vi "KickForceIRL.vi"(0 "Game in":refnum<class "Game.lvclass">, 1 "KickValueTest":T1={"ForceValue"={"delta_kick"=0.0, "kick_min"=1.0, "kick_max"=0.0}, "BallValue"={"delta_ball"=0.0, "v_min_ball"=1.0, "v_max_ball"=0.0}, "Samples"=0.0, "Start"=FALSE, "id"=0, "RobotStopKick"=FALSE}, 3 "error in (no error)":errorcluster) -> (7 "Game out":refnum<class "Game.lvclass">, 8 "TestTeam":refnum<class "Ally.lvclass">, 10 "error out":errorcluster)   [LabVIEW 2021, in "Game.lvclass"]
uses:
  Game.lvclass
  Ally_class/Ally.lvclass
  KickValueTest/KickValuetest.ctl
  KickValueTest/KickValue.ctl
  KickValueTest/BallValue.ctl
  KickForceIRL/KickForceIRLstates.ctl
  Game.lvclass/Game.ctl
  Object_class/Object.lvclass/Object.ctl
  Ball_class/Ball.lvclass/Ball.ctl
  Team_class/Team.lvclass/Team.ctl
  RobotFeedback/RobotFeedback.lvclass/RobotFeedback.ctl
  Robot_class/Robot.lvclass/Robot.ctl
  RobotFeedback/Read id.vi
  RobotFeedback/Read dribblerContactToBall.vi
  <vilib>/Analysis/baseanly.llb/Unit Vector (DBL).vi
  Robot_class/Write kick_x.vi
  Robot_class/Write dest_x.vi
  Robot_class/Write dest_y.vi
  Read BallRef.vi
  Read FieldRef.vi
  Read AllyRef.vi
  Read Utilities.lvclass.vi
  Read TestTeam.vi
  Read RobotsFeedback.vi
  Team_class/Read RobotRef.vi
  Object_class/Read position(x,y).vi
  Ball_class/Read v_x.vi
  Ball_class/Read v_y.vi
  Object_class/Read x.vi
  Object_class/Read y.vi
  Team_class/Write RobotRef.vi
  Ball_class/Ball.lvclass
  Robot_class/Robot.lvclass
  <vilib>/Analysis/1siggen.llb/Ramp Pattern by Delta.vi
  Field_class/Field.lvclass
  Utilities_class/Utilities.lvclass
  RobotFeedback/RobotFeedback.lvclass
  <vilib>/Analysis/NI_AALBase.lvlib
panel:
  out "appended array":dbl[][](array[numeric])
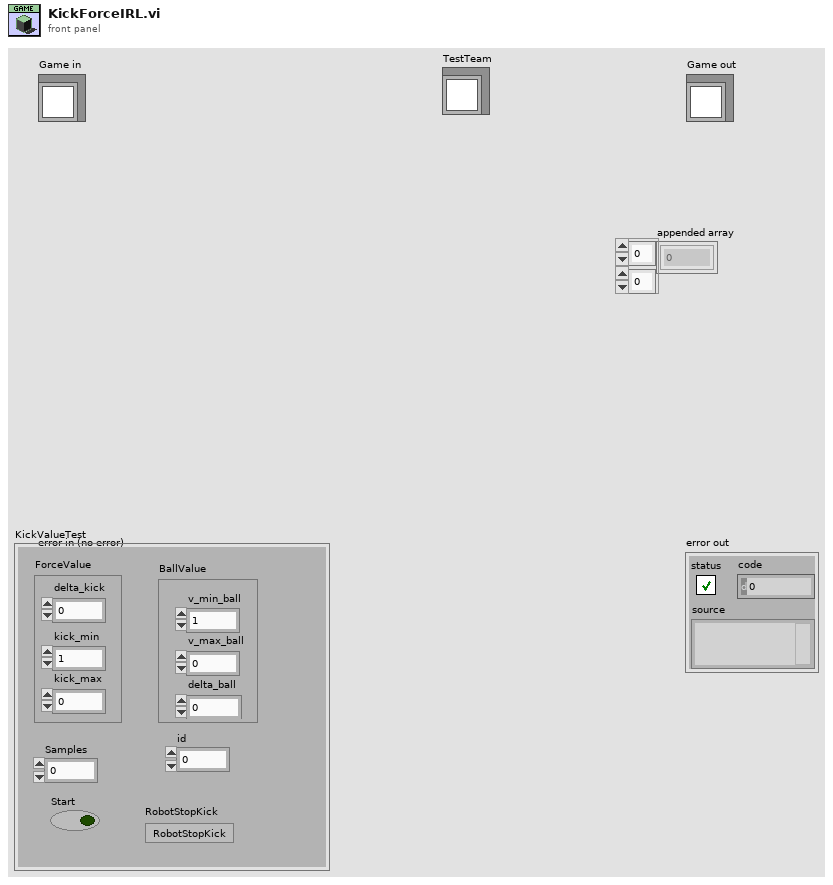
[diagram p1: front panel]
types:
  T1 = typedef "KickValuetest.ctl" = cluster{"ForceValue":T2, "BallValue":T3, "Samples":dbl, "Start":bool, "id":i32, "RobotStopKick":bool}
  T2 = typedef "Game.lvclass/KickValue.ctl" = cluster{"delta_kick":dbl, "kick_min":dbl, "kick_max":dbl}
  T3 = typedef "Game.lvclass/BallValue.ctl" = cluster{"delta_ball":dbl, "v_min_ball":dbl, "v_max_ball":dbl}
  T4 = typedef "Game.lvclass/KickForceIRLstates.ctl" = enum16{"Ball positioning", "Start count time", "Kicking ball", "Waiting ball v=0", "Saiving kick force, time and distance", "Finish"}
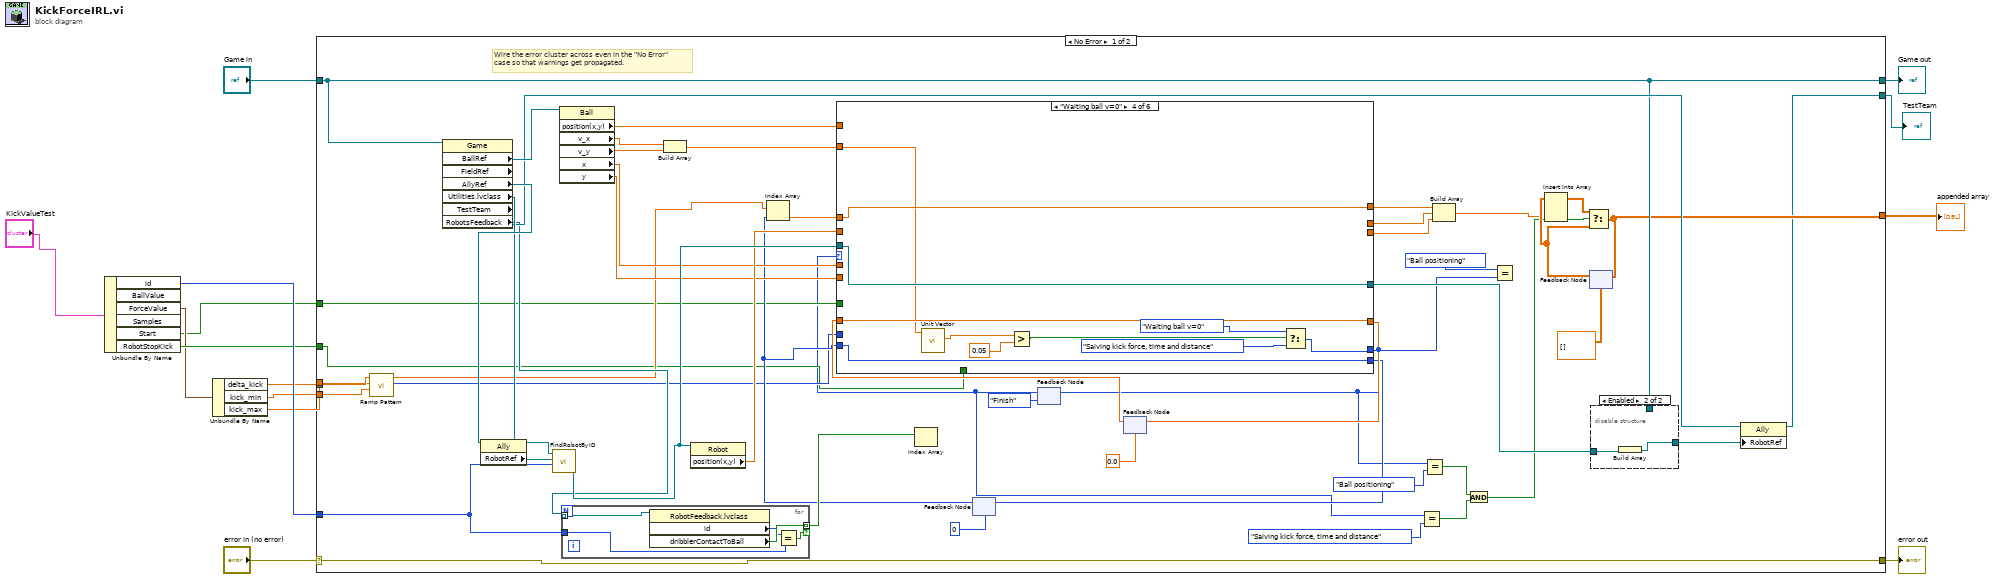
[diagram p0: block diagram]
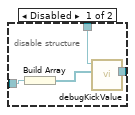
[diagram p2: hidden frame]
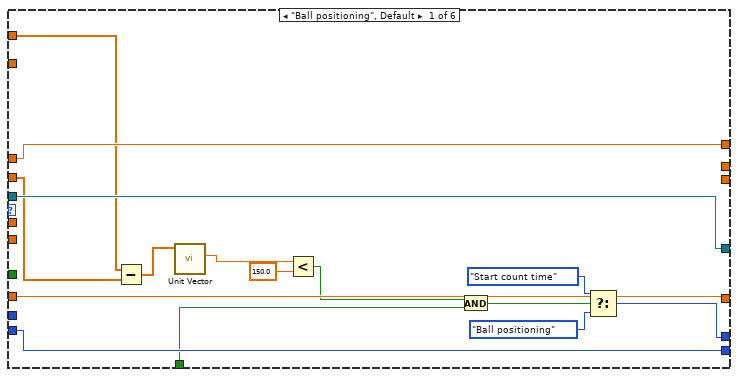
[diagram p3: hidden frame]
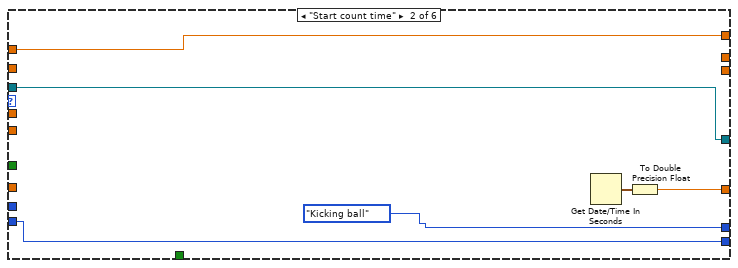
[diagram p4: hidden frame]
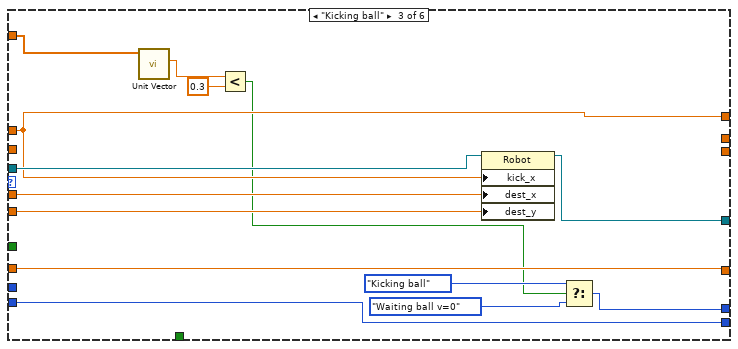
[diagram p5: hidden frame]
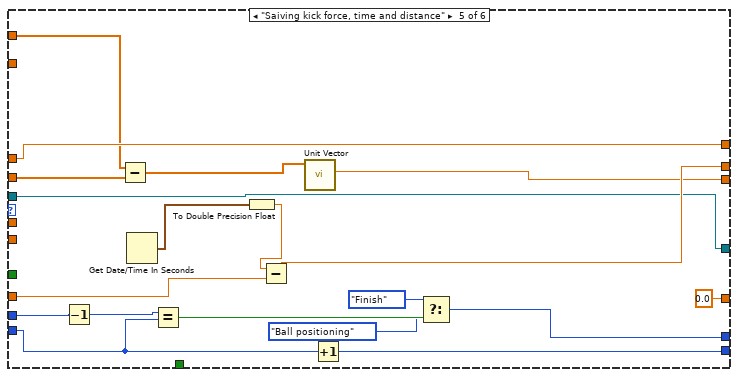
[diagram p6: hidden frame]
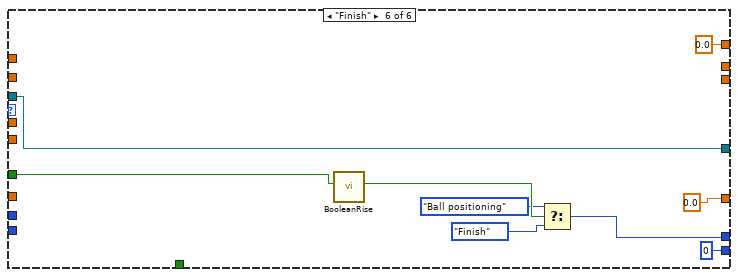
[diagram p7: hidden frame]
diagram:
  n1 = Unbundle By Name("KickValueTest") -> ("id"=w8:i32, "ForceValue"=w6:T2, "Start"=w2:bool, "RobotStopKick"=w7:bool)  [unwired: 2 out]
  n2 = Unbundle By Name(w6) -> ("delta_kick"=w5:dbl, "kick_min"=w4:dbl, "kick_max"=w3:dbl)
  n3 = case shown="No Error" "error in (no error)" {
    selector: "error in (no error)" -> [w66 w153]
    tunnel: [w66 w153] -> w13
    tunnel: [w59 w152] -> w11
    tunnel: "Game in" -> [w59 w152]
    tunnel: [w32 _] -> w10
    tunnel: w8 -> [w40 _]
    tunnel: w7 -> [w25 _]
    tunnel: [w42 _] -> w1
    tunnel: w5 -> [w36 _]
    tunnel: w4 -> [w35 _]
    tunnel: w3 -> [w34 _]
    tunnel: w2 -> [w28 _]
    frame No Error {
      # "Wire the error cluster across even in the \"No Error\"\ncase so that warnings get propagated."
      n4 = call-poly <vilib>:"Ramp Pattern.vi"("start"=w35, "end"=w34, "delta"=w36) -> ("samples"=w30:i32, "Ramp Pattern"=w29:dbl[])  [unwired: 6 in, 1 out]
      n5 = property class="Game" props=["BallRef", "FieldRef", "AllyRef", "Utilities.lvclass", "TestTeam", "RobotsFeedback"](reference=w59) -> ("BallRef"=w65:refnum<class "Ball.lvclass">, "AllyRef"=w64:refnum<class "Ally.lvclass">, "Utilities.lvclass"=w62:refnum<class "Utilities.lvclass">, "TestTeam"=w61:refnum<class "Ally.lvclass">, "RobotsFeedback"=w41:refnum<class "RobotFeedback.lvclass">[])  [unwired: 1 in, 3 out]
      n6 = property class="Ally"(reference=w64) -> ("RobotRef"=w63:refnum<class "Robot.lvclass">[])  [unwired: 1 in, 2 out]
      n7 = call "FindRobotByID.vi"("id"=w40, "RobotRef"=w63, "Utilities in"=w62) -> ("Robot"=w58:refnum<class "Robot.lvclass">)  [unwired: 5 in, 3 out]
      n8 = property class="Ball"(reference=w65) -> ("position(x,y)"=w45:dbl[], "v_x"=w51:dbl, "v_y"=w50:dbl, "x"=w38:dbl, "y"=w37:dbl)  [unwired: 1 in, 2 out]
      n9 = for {
        tunnel: w41 -> [w77] mode=indexing
        tunnel: w40 -> [w74]
        tunnel: [w76] -> w39 mode=indexing if=w73
        n10 = property class="RobotFeedback.lvclass"(reference=w77) -> ("id"=w75:i32, "dribblerContactToBall"=w76:bool)  [unwired: 1 in, 2 out]
        n11 = Equal?(x=w75, y=w74) -> (x = y?=w73:bool)
      }
      n12 = Build Array(w51, w50) -> (w49:dbl[])
      n13 = property class="Robot"(reference=w58) -> ("position(x,y)"=w46:dbl[])  [unwired: 1 in, 2 out]
      n14 = Index Array(array=w39) -> ()  [unwired: 1 in, 1 out]
      n15 = feedback #1(0) -> (w31:i32)
      n16 = Index Array(array=w29, index=w31) -> (element=w47:dbl)
      n17 = feedback #2(KickForceIRLstates."Finish" ("t")) -> (w21:T4)
      n18 = feedback #3(0.0) -> (w56:dbl)
      n19 = case shown="\"Waiting ball v=0\"" w21 {
        tunnel: [w78 KickForceIRLstates."Kicking ball" w103 w117 w129 w143] -> w24
        tunnel: [w92 w96 w112 w123 0.0 0.0] -> w57
        tunnel: w56 -> [w92 _ w112 w123 w142 _]
        tunnel: [_ _ _ _ w139 _] -> w55
        tunnel: w58 -> [w89 w93 w111 w115 w133 w150]
        tunnel: [w91 w95 w110 w122 w137 0] -> w53
        tunnel: w31 -> [w91 w95 w110 w122 w128 _]
        tunnel: w49 -> [_ _ w102 w114 _ _]
        tunnel: [w90 w94 w109 w116 w136 0.0] -> w48
        tunnel: w47 -> [w90 w94 w109 w116 w136 _]
        tunnel: w46 -> [w87 _ _ _ w135 _]
        tunnel: w45 -> [w88 _ _ _ w134 _]
        tunnel: [w89 w93 w108 w115 w133 w150] -> w33
        tunnel: w25 -> [w82 _ _ _ _ _]
        tunnel: w38 -> [_ _ w107 _ _ _]
        tunnel: w37 -> [_ _ w106 _ _ _]
        tunnel: w30 -> [_ _ _ _ w127 _]
        tunnel: w28 -> [_ _ _ _ _ w147]
        tunnel: [_ _ _ _ w124 _] -> w17
        frame "Ball positioning", Default {
          n20 = Subtract(x=w88, y=w87) -> (x-y=w86:dbl[])
          n21 = call-poly <vilib>:"Unit Vector.vi"("Input Vector"=w86) -> ("norm"=w85:dbl)  [unwired: 8 in, 2 out]
          n22 = Less?(x=w85, y=150.0) -> (x < y?=w83:bool)
          n23 = And(x=w83, y=w82) -> (x .and. y?=w81:bool)
          n24 = Select(t=KickForceIRLstates."Start count time", s=w81, f=KickForceIRLstates."Ball positioning") -> (s? t:f=w78:T4)
        }
        frame "Start count time" {
          n25 = Get Date/Time In Seconds() -> (seconds since 1Jan1904=w97:timestamp)
          n26 = To Double Precision Float(number=w97) -> (double precision float=w96:dbl)
        }
        frame "Kicking ball" {
          n27 = call-poly <vilib>:"Unit Vector.vi"("Input Vector"=w102) -> ("norm"=w101:dbl)  [unwired: 8 in, 2 out]
          n28 = Less?(x=w101, y=0.3) -> (x < y?=w99:bool)
          n29 = property class="Robot"(reference=w111, "kick_x"=w109, "dest_x"=w107, "dest_y"=w106) -> (reference out=w108:refnum<class "Robot.lvclass">)  [unwired: 1 in, 1 out]
          n30 = Select(t=KickForceIRLstates."Kicking ball", s=w99, f=KickForceIRLstates."Waiting ball v=0") -> (s? t:f=w103:T4)
        }
        frame "Waiting ball v=0" {
          n31 = call-poly <vilib>:"Unit Vector.vi"("Input Vector"=w114) -> ("norm"=w113:dbl)  [unwired: 8 in, 2 out]
          n32 = Greater?(x=w113, y=0.05) -> (0:w118:bool)
          n33 = Select(t=KickForceIRLstates."Waiting ball v=0", s=w118, f=KickForceIRLstates."Saiving kick force, time and distance") -> (s? t:f=w117:T4)
        }
        frame "Saiving kick force, time and distance" {
          n34 = Decrement(x=w127) -> (x-1=w126:i32)
          n35 = Subtract(x=w134, y=w135) -> (x-y=w125:dbl[])
          n36 = Get Date/Time In Seconds() -> (seconds since 1Jan1904=w141:timestamp)
          n37 = Equal?(x=w126, y=w128) -> (x = y?=w132:bool)
          n38 = To Double Precision Float(number=w141) -> (double precision float=w140:dbl)
          n39 = Subtract(x=w140, y=w142) -> (x-y=w139:dbl)
          n40 = call-poly <vilib>:"Unit Vector.vi"("Input Vector"=w125) -> ("norm"=w124:dbl)  [unwired: 8 in, 2 out]
          n41 = Increment(x=w128) -> (x+1=w137:i32)
          n42 = Select(t=KickForceIRLstates."Finish", s=w132, f=KickForceIRLstates."Ball positioning") -> (s? t:f=w129:T4)
        }
        frame "Finish" {
          n43 = call "BooleanRise.vi"("Boolean in"=w147) -> ("Boolean"=w146:bool)  [unwired: 8 in, 2 out]
          n44 = Select(t=KickForceIRLstates."Ball positioning", s=w146, f=KickForceIRLstates."Finish" ("t")) -> (s? t:f=w143:T4)
        }
      }
      n45 = feedback-in #1(w53) -> ()
      n46 = feedback-in #2(w24) -> ()
      n47 = feedback-in #3(w57) -> ()
      n48 = Equal?(x=w21, y=KickForceIRLstates."Saiving kick force, time and distance" ("x")) -> (x = y?=w19:bool)
      n49 = Equal?(x=w24, y=KickForceIRLstates."Ball positioning" ("x")) -> (x = y?=w20:bool)
      n50 = Build Array(w48, w55, w17) -> (w15:dbl[])
      n51 = And(x=w20, y=w19) -> (x .and. y?=w18:bool)
      n52 = Equal?(x=KickForceIRLstates."Ball positioning", y=w24) -> ()  [unwired: 1 out]
      n53 = feedback #4(dbl[][] [] ("appended array")) -> (w43:dbl[][])
      n54 = Insert Into Array(array=w43, new element=w15) -> (w44:dbl[][])  [unwired: 2 in]
      n55 = Select(t=w44, s=w18, f=w43) -> (s? t:f=w42:dbl[][])
      n56 = feedback-in #4(w42) -> ()
      n57 = disable-structure shown="Enabled" {
        disable-tunnel: [w70 w71] -> w60
        disable-tunnel: w59 -> [w68 _]
        disable-tunnel: w33 -> [w67 w72]
        frame Disabled {
          n58 = Build Array(w67) -> (w69:refnum<class "Robot.lvclass">[])
          n59 = call "debugKickValue.vi"("RoboRefArray in"=w69, "Game in"=w68) -> ("RoboRefArray out"=w70:refnum<class "Robot.lvclass">[])  [unwired: 7 in, 2 out]
        }
        frame Enabled {
          n60 = Build Array(w72) -> (w71:refnum<class "Robot.lvclass">[])
        }
      }
      n61 = property class="Ally"(reference=w61, "RobotRef"=w60) -> (reference out=w32:refnum<class "Ally.lvclass">)  [unwired: 1 in, 1 out]
    }
    frame Error {
    }
  }
  "error out" <- w13
  "Game out" <- w11
  "TestTeam" <- w10
  "appended array" <- w1
